vi "svl_Check Data Valid [SLM].vi"(4 "decimation factor":i32=1 min=1 step=1, 5 "time constant [ms]":dbl=125.0 format="%.2f", 6 "integration time [s]":dbl=1.0 format="%.2f", 7 "exponential mode":enum16{"Slow", "Fast", "Impulse", "Custom"}(ring)=enum."Fast", 8 "error in (no error)":errorcluster, 9 "restart averaging (F)":bool, 10 "Level Analysis":T4(ring), 11 "scaled signal [EU]":waveform(dbl)) -> (0 "error out":errorcluster, 1 "processing state":T5(ring), 2 "channel info":T1 {"pregain" format="%.2f"; "weighting filter" items=["Linear", "A-weighting", "B-weighting", "C-weighting", "ITU-R 468-4", "Dolby", "CCITT", "C-message", "Wb", "Wc", "Wd", "We", "Wf", "Wh", "Wj", "Wk", "Wm", "AES17 20 kHz lowpass", "AES17 40 kHz lowpass", "AES17 20 kHz highpass", "AES17 40 kHz highpass"]; "dB reference" format="%^.1e"; "engineering units" items=["custom..."=0, "V"=1, "A"=21, "C"=30, "pC"=31, "s"=32, "-"=29, "Pa"=2, "N"=20, "g"=3, "m/s^2"=4, "m/s"=5, "m"=6, "mm/s"=12, "mm"=13, "micron/s"=14, "micron"=15, "in/s^2"=7, "in/s"=8, "in"=9, "mil/s"=10, "mil"=11, "rad/s^2"=16, "rad/s"=17, "rad"=18, "deg/s^2"=26, "deg/s"=27, "deg"=28, "RPM"=22, "cycle/s^2"=23, "Hz"=24, "cycle"=25, "strain"=19]; "sensor sensitivity" format="%#_5f"}, 3 "dup scaled signal [EU]":waveform(dbl))   [LabVIEW 2017]
uses:
  <vilib>/addons/_NISVFA/_Shared subVIs/Controls/svc_Channel Info.ctl
  <vilib>/addons/_NISVFA/_Shared subVIs/Controls/svc_Engineering Units Text Ring.ctl
  <vilib>/addons/_NISVFA/_Shared subVIs/Controls/svc_Weighting Filter Text Ring.ctl
  <vilib>/addons/_NISVFA/_Shared subVIs/Common/svc_Check for Waveform Parameter Continuity (no state).vi
  <vilib>/addons/_NISVFA/_Shared subVIs/Common/svc_Get SV Channel Info.vi
  <vilib>/addons/_NISVFA/_Shared subVIs/Common/svc_Engineering Units to Unit Label.vi
  <vilib>/addons/_NISVFA/_Shared subVIs/Common/svc_Unit Label to Engineering Units.vi
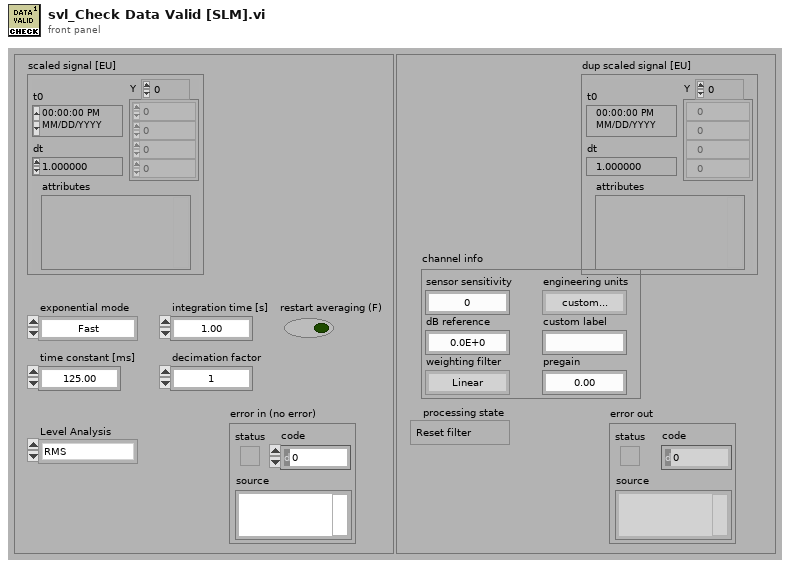
[diagram p1: front panel]
types:
  T1 = typedef "svc_Channel Info.ctl" = cluster{"sensor sensitivity":dbl, "engineering units":T2, "dB reference":dbl, "custom label":string, "weighting filter":T3, "pregain":dbl}
  T2 = typedef "svc_Engineering Units Text Ring.ctl" = u16
  T3 = typedef "svc_Weighting Filter Text Ring.ctl" = u16
  T4 = enum16{"RMS", "Running RMS", "Exp avg  ", "Dec exp avg ", "Peak", "Crest"}
  T5 = enum16{"Reset filter", "Restart averaging", "Continue processing"}
  T6 = cluster{"dt":bool, "t0 continuity":bool, "array length":bool, "channel info":bool, "name":bool}
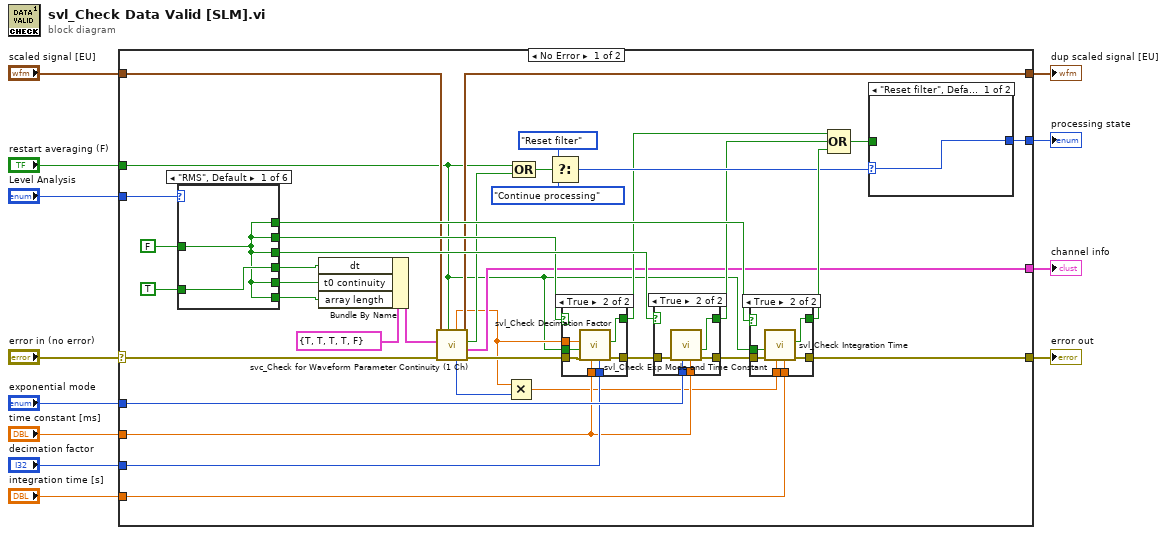
[diagram p0: block diagram]
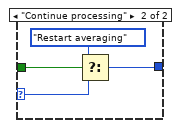
[diagram p2: hidden frame]
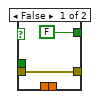
[diagram p3: hidden frame]
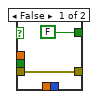
[diagram p4: hidden frame]
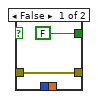
[diagram p5: hidden frame]
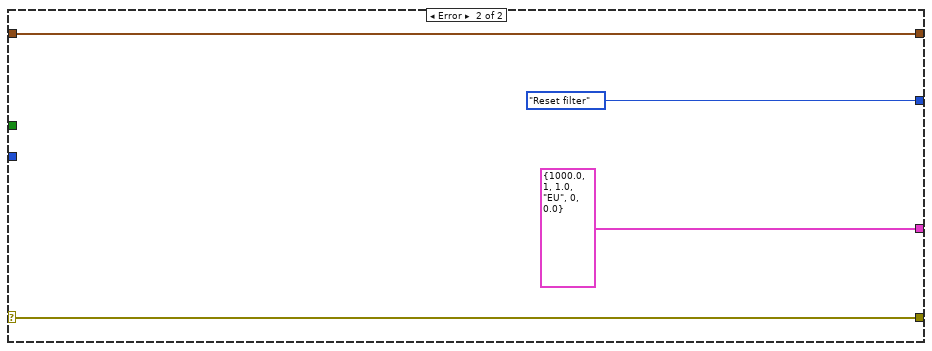
[diagram p11: hidden frame]
diagram:
  n1 = case shown="No Error" "error in (no error)" {
    selector: "error in (no error)" -> [w21 w93]
    tunnel: [w29 w93] -> w10
    tunnel: "restart averaging (F)" -> [w14 _]
    tunnel: "time constant [ms]" -> [w35 _]
    tunnel: [w41 T5."Reset filter" ("processing state")] -> w7
    tunnel: "Level Analysis" -> [w48 _]
    tunnel: "integration time [s]" -> [w47 _]
    tunnel: "decimation factor" -> [w46 _]
    tunnel: "exponential mode" -> [w49 _]
    tunnel: "scaled signal [EU]" -> [w20 w90]
    tunnel: [w19 T1 {"sensor sensitivity"=1000.0, "engineering units"=1, "dB reference"=1.0, "custom label"="EU", "weighting filter"=0, "pregain"=0.0} ("channel info")] -> w2
    tunnel: [w18 w90] -> w1
    frame No Error {
      n2 = case shown="\"RMS\", Default" w48 {
        tunnel: [w79 w82 w84 w86 w87 w88] -> w40
        tunnel: [w79 w82 w83 w86 w87 w88] -> w39
        tunnel: [w79 w81 w83 w85 w87 w88] -> w38
        tunnel: [w79 w81 w83 w85 w87 w88] -> w23
        tunnel: [w79 w81 w84 w86 w87 w88] -> w33
        tunnel: [w80 w81 w84 w86 w87 w89] -> w32
        tunnel: FALSE -> [w79 w82 w83 w85 w87 w88]
        tunnel: TRUE -> [w80 w81 w84 w86 _ w89]
        frame "RMS", Default {
        }
        frame "Running RMS" {
        }
        frame "Exp avg  " {
        }
        frame "Dec exp avg " {
        }
        frame "Peak" {
        }
        frame "Crest" {
        }
      }
      n3 = Bundle By Name(cluster=T6 {"dt"=TRUE, "t0 continuity"=TRUE, "array length"=TRUE, "channel info"=TRUE, "name"=FALSE} ("checks for channel parameter change"), "dt"=w32, "t0 continuity"=w33, "array length"=w23) -> (w34:T6)
      n4 = call <vilib>:"svc_Check for Waveform Parameter Continuity (1 Ch).vi"("restart averaging (F)"=w14, "error in (no error)"=w21, "checks for channel parameter change"=w34, "scaled signal [EU]"=w20) -> ("error out"=w28:errorcluster, "channel info"=w19:T1, "waveform parameter changed"=w22:bool, "dup scaled signal [EU]"=w18:waveform(dbl), "array length"=w16:i32, "dt"=w17:dbl)  [unwired: 2 in]
      n5 = Multiply(x=w17, y=w16) -> (x*y=w15:dbl)
      n6 = Compound Arithmetic op=OR(w14, w22) -> (w36:bool)
      n7 = Select(t=T5."Reset filter" ("processing state"), s=w36, f=T5."Continue processing" ("processing state")) -> (s? t:f=w42:T5)
      n8 = case shown="True" w39 {
        tunnel: w28 -> [w64 w71]
        tunnel: [w64 w70] -> w31
        tunnel: w35 -> [_ w68]
        tunnel: w46 -> [_ w67]
        tunnel: [FALSE ("parameter has changed") w69] -> w26
        tunnel: w17 -> [_ w66]
        tunnel: w14 -> [_ w65]
        frame False {
        }
        frame True {
          n9 = call <vilib>:"svl_Check Decimation Factor.vi"("decimation factor"=w67, "time constant [ms]"=w68, "error in (no error)"=w71, "restart averaging (F)"=w65, "dt"=w66) -> ("error out"=w70:errorcluster, "parameter has changed"=w69:bool)  [unwired: 5 in]
        }
      }
      n10 = case shown="True" w40 {
        tunnel: w49 -> [_ w78]
        tunnel: w31 -> [w73 w74]
        tunnel: [w73 w77] -> w30
        tunnel: [FALSE w75] -> w27
        tunnel: w35 -> [_ w76]
        frame False {
        }
        frame True {
          n11 = call <vilib>:"svl_Check Exp Mode and Time Constant.vi"("time constant [ms]"=w76, "exponential mode"=w78, "error in (no error)"=w74) -> ("error out"=w77:errorcluster, "parameter has changed"=w75:bool)  [unwired: 7 in]
        }
      }
      n12 = case shown="True" w38 {
        tunnel: w30 -> [w56 w62]
        tunnel: [w56 w61] -> w29
        tunnel: w47 -> [_ w59]
        tunnel: [FALSE ("parameter has changed") w60] -> w45
        tunnel: w15 -> [_ w58]
        tunnel: w14 -> [_ w57]
        frame False {
        }
        frame True {
          n13 = call <vilib>:"svl_Check Integration Time.vi"("integration time"=w59, "acquisition period"=w58, "error in (no error)"=w62, "restart averaging (F)"=w57) -> ("error out"=w61:errorcluster, "parameter has changed"=w60:bool)  [unwired: 5 in, 1 out]
        }
      }
      n14 = Compound Arithmetic op=OR(w26, w27, w45) -> (w37:bool)
      n15 = case shown="\"Reset filter\", Default" w42 {
        selector: w42 -> [w50 w53]
        tunnel: w37 -> [_ w54]
        tunnel: [w50 w51] -> w41
        frame "Reset filter", Default {
        }
        frame "Continue processing" {
          n16 = Select(t=T5."Restart averaging" ("processing state"), s=w54, f=w53) -> (s? t:f=w51:T5)
        }
      }
    }
    frame Error {
      (unwired) TRUE ("t0 changed")
    }
  }
  "error out" <- w10
  "processing state" <- w7
  "dup scaled signal [EU]" <- w1
  "channel info" <- w2
